vi "attribute_get_cache_or_default_value.vi"(7 "Attribute":T1={"Identifier"="", "Descriptive Name"="", "Data Type"=enum."Integer 32", "Command"="", "Access"=enum."Read/Write", "Range Table"="", "Read Callback"="", "Write Callback"="", "Supported Models"="", "Instrument Options"="", "Index"=0, "OPC Wait"=FALSE, "No Status Check"=FALSE, "Cache Only"=FALSE}, 8 "error in":errorcluster caption="error in (no error)", 11 "VISA resource name":refnum<visa-resource-name>) -> (0 "error out":errorcluster, 1 "Int32 out":i32, 2 "Double out":dbl, 3 "VISA resource name out":refnum<visa-resource-name>, 4 "String out":string, 5 "Int64 out":i64, 6 "Boolean out":bool, 9 "Exists in cache":bool)   [LabVIEW 2022 SP3, in "hmp4000_rsidr_core.lvlib"]
uses:
  hmp4000_rsidr_core.lvlib
  type_Attribute.ctl
  type_Attribute_Data_Type.ctl
  type_ReadWriteAccess.ctl
  _type_Operation_Fgv_RangeTable.ctl
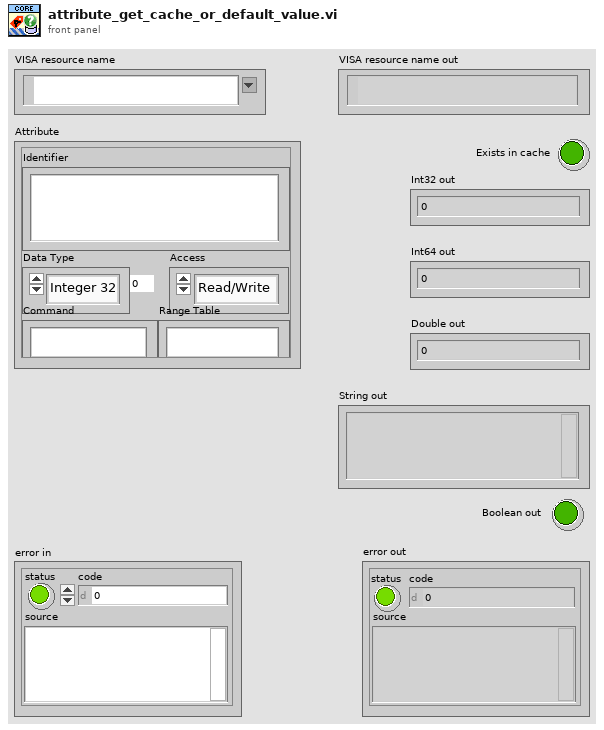
[diagram p1: front panel]
types:
  T1 = typedef "hmp4000_rsidr_core.lvlib/type_Attribute.ctl" = cluster{"Identifier":string, "Descriptive Name":string, "Data Type":T2, "Command":string, "Access":T3, "Range Table":string, "Read Callback":string, "Write Callback":string, "Supported Models":string, "Instrument Options":string, "Index":i32, "OPC Wait":bool, "No Status Check":bool, "Cache Only":bool}
  T2 = typedef "hmp4000_rsidr_core.lvlib/type_Attribute_Data_Type.ctl" = enum16{"Integer 32", "Double", "String", "Boolean", "None", "Integer 64", "RawString"}
  T3 = typedef "hmp4000_rsidr_core.lvlib/type_ReadWriteAccess.ctl" = enum16{"Read Only", "Write Only", "Read/Write"}
  T4 = typedef "hmp4000_rsidr_core.lvlib/_type_Operation_Fgv_RangeTable.ctl" = enum16{"Initialize", "Check", "Coerce", "Get Command String", "Get Numeric Value", "Get Default Value", "Get Range Table Type"}
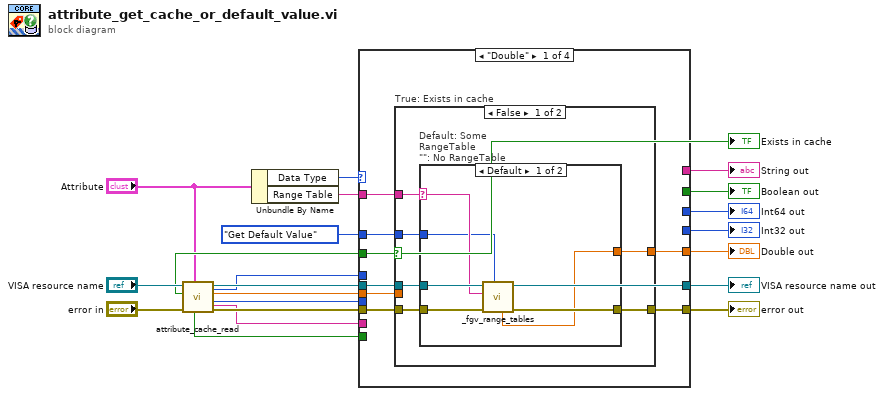
[diagram p0: block diagram]
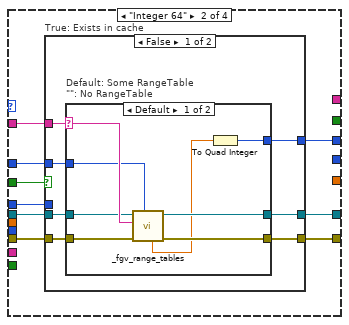
[diagram p4: hidden frame]
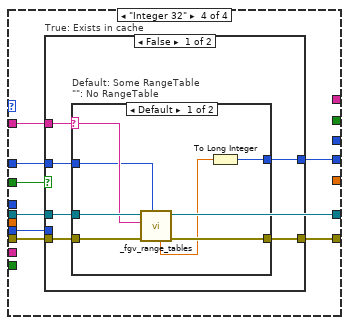
[diagram p8: hidden frame]
diagram:
  n1 = call "attribute_cache_read.vi"("Attribute"="Attribute", "error in"="error in", "VISA resource name"="VISA resource name") -> ("error out"=w13:errorcluster, "Int32 out"=w7:i32, "Double out"=w10:dbl, "VISA resource name out"=w12:refnum<visa-resource-name>, "String out"=w6:string, "Int64 out"=w9:i64, "Boolean out"=w4:bool, "Exists in cache"=w11:bool)  [unwired: 1 in]
  "Exists in cache" <- w11
  n2 = Unbundle By Name("Attribute") -> ("Data Type"=w18:T2, "Range Table"=w8:string)
  n3 = case shown="\"Double\"" w18 {
    tunnel: w13 -> [w27 w49 w77 w82]
    tunnel: w12 -> [w23 w47 w76 w79]
    tunnel: [w29 w53 w77 w85] -> w21
    tunnel: [w23 w46 w76 w79] -> w20
    tunnel: [w28 _ _ _] -> w19
    tunnel: [_ _ _ w84] -> w17
    tunnel: [_ w52 _ _] -> w16
    tunnel: w11 -> [w25 w50 _ w80]
    tunnel: w10 -> [w26 _ _ _]
    tunnel: w9 -> [_ w51 _ _]
    tunnel: w8 -> [w24 w48 _ w83]
    tunnel: w7 -> [_ _ _ w81]
    tunnel: w6 -> [_ _ w75 _]
    tunnel: [_ _ w75 _] -> w5
    tunnel: w4 -> [_ _ w74 _]
    tunnel: [_ _ w74 _] -> w3
    tunnel: _type_Operation_Fgv_RangeTable."Get Default Value" ("Operation") -> [w22 w45 _ w78]
    frame "Double" {
      n4 = case "True: Exists in cache" shown="False" w25 {
        tunnel: w27 -> [w34 w44]
        tunnel: w26 -> [_ w43]
        tunnel: [w33 w44] -> w29
        tunnel: w24 -> [w35 _]
        tunnel: [w32 w43] -> w28
        tunnel: w23 -> [w31 _]
        tunnel: w22 -> [w30 _]
        frame False {
          n5 = case "Default: Some RangeTable\n\"\": No RangeTable" shown="Default" w35 {
            selector: w35 -> [w39 _]
            tunnel: w34 -> [w41 w42]
            tunnel: [w40 w42] -> w33
            tunnel: [w36 _] -> w32
            tunnel: w31 -> [w38 _]
            tunnel: w30 -> [w37 _]
            frame Default {
              n6 = call "_fgv_range_tables.vi"("Operation"=w37, "error in"=w41, "Range Table ID in"=w39, "VISA resource name"=w38) -> ("error out"=w40:errorcluster, "Numeric Value out"=w36:dbl)  [unwired: 3 in, 3 out]
            }
            frame "" {
            }
          }
        }
        frame True {
        }
      }
    }
    frame "Integer 64" {
      n7 = case "True: Exists in cache" shown="False" w50 {
        tunnel: w49 -> [w59 w73]
        tunnel: w51 -> [_ w72]
        tunnel: [w58 w73] -> w53
        tunnel: w48 -> [w60 _]
        tunnel: [w57 w72] -> w52
        tunnel: w47 -> [w56 w71]
        tunnel: [w55 w71] -> w46
        tunnel: w45 -> [w54 _]
        frame False {
          n8 = case "Default: Some RangeTable\n\"\": No RangeTable" shown="Default" w60 {
            selector: w60 -> [w66 _]
            tunnel: w59 -> [w68 w70]
            tunnel: [w67 w70] -> w58
            tunnel: [w61 _] -> w57
            tunnel: w56 -> [w65 w69]
            tunnel: [w64 w69] -> w55
            tunnel: w54 -> [w63 _]
            frame Default {
              n9 = call "_fgv_range_tables.vi"("Operation"=w63, "error in"=w68, "Range Table ID in"=w66, "VISA resource name"=w65) -> ("error out"=w67:errorcluster, "VISA resource name out"=w64:refnum<visa-resource-name>, "Numeric Value out"=w62:dbl)  [unwired: 3 in, 2 out]
              n10 = To Quad Integer(1:w62) -> (0:w61:i64)
            }
            frame "" {
            }
          }
        }
        frame True {
        }
      }
    }
    frame Default {
    }
    frame "Integer 32" {
      n11 = case "True: Exists in cache" shown="False" w80 {
        tunnel: w82 -> [w91 w101]
        tunnel: w81 -> [_ w100]
        tunnel: [w90 w101] -> w85
        tunnel: [w89 w100] -> w84
        tunnel: w83 -> [w88 _]
        tunnel: w79 -> [w87 _]
        tunnel: w78 -> [w86 _]
        frame False {
          n12 = case "Default: Some RangeTable\n\"\": No RangeTable" shown="Default" w88 {
            selector: w88 -> [w96 _]
            tunnel: w91 -> [w98 w99]
            tunnel: [w97 w99] -> w90
            tunnel: [w92 _] -> w89
            tunnel: w87 -> [w95 _]
            tunnel: w86 -> [w94 _]
            frame Default {
              n13 = call "_fgv_range_tables.vi"("Operation"=w94, "error in"=w98, "Range Table ID in"=w96, "VISA resource name"=w95) -> ("error out"=w97:errorcluster, "Numeric Value out"=w93:dbl)  [unwired: 3 in, 3 out]
              n14 = To Long Integer(number=w93) -> (32bit integer=w92:i32)
            }
            frame "" {
            }
          }
        }
        frame True {
        }
      }
    }
  }
  "VISA resource name out" <- w20
  "error out" <- w21
  "Int64 out" <- w16
  "Int32 out" <- w17
  "Double out" <- w19
  "String out" <- w5
  "Boolean out" <- w3
